vi "_Counter-Decrement.vi"(6 "LIBNAME":string, 7 "VI Refnum":refnum<vi>, 8 "error in (no error)":errorcluster, 9 "force destroy?(F)":bool, 11 "StopSignal":T2) -> (0 "error out":errorcluster, 1 "cache":T1)   [LabVIEW 2017, in "StopSignal.lvlib"]
uses:
  StopSignal.lvlib
  Typedef/StopSignal.ctl
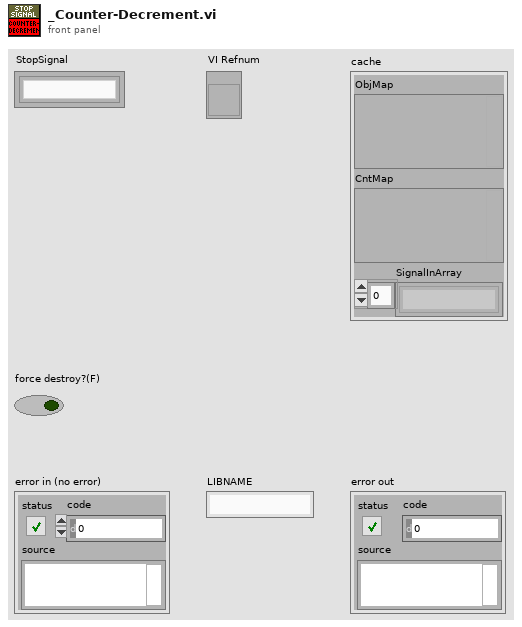
[diagram p1: front panel]
types:
  T1 = cluster{"ObjMap":variant, "CntMap":variant, "SignalInArray":string[]}
  T2 = typedef "StopSignal.lvlib/StopSignal.ctl" = refnum<k1>
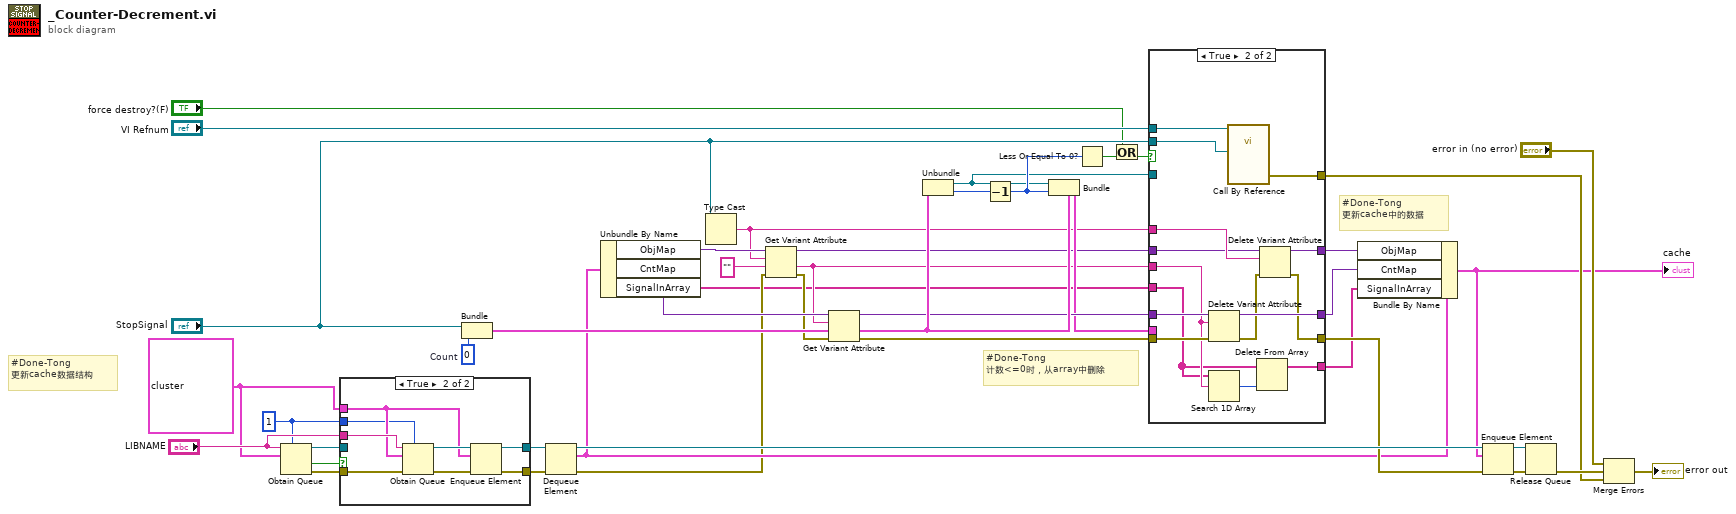
[diagram p0: block diagram]
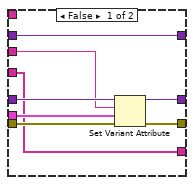
[diagram p2: hidden frame]
diagram:
  w4 = T1 {"ObjMap"=variant, "CntMap"=variant, "SignalInArray"=[]}
  w20 = 1 ("max queue size (-1, unlimited)")
  w30 = 0  # Count
  # "#Done-Tong\n更新cache中的数据"
  # "#Done-Tong\n计数<=0时，从array中删除"
  # "#Done-Tong\n更新cache数据结构"
  n1 = Obtain Queue(max queue size (-1, unlimited)=w20, name (unnamed)="LIBNAME", element data type=w4) -> (queue out=w41:refnum<queue>, created new?=w43:bool, error out=w42:errorcluster)  [unwired: 2 in]
  n2 = case shown="True" w43 {
    tunnel: w42 -> [w45 w52]
    tunnel: w41 -> [w46 _]
    tunnel: w4 -> [_ w48]
    tunnel: [w45 w54] -> w40
    tunnel: [w46 w53] -> w39
    tunnel: "LIBNAME" -> [_ w49]
    tunnel: w20 -> [_ w47]
    frame False {
    }
    frame True {
      n3 = Obtain Queue(max queue size (-1, unlimited)=w47, name (unnamed)=w49, element data type=w48, error in (no error)=w52) -> (queue out=w50:refnum<queue>, error out=w51:errorcluster)  [unwired: 1 in, 1 out]
      n4 = Enqueue Element(queue=w50, element=w48, error in (no error)=w51) -> (queue out=w53:refnum<queue>, error out=w54:errorcluster)  [unwired: 1 in, 1 out]
    }
  }
  n5 = Bundle("StopSignal"="StopSignal", "Count"=w30) -> (w29:cluster{"StopSignal":T2, "Count":i32})  [unwired: 1 in]
  n6 = Dequeue Element(queue=w39, error in (no error)=w40) -> (queue out=w35:refnum<queue>, element=w18:T1, error out=w9:errorcluster)  [unwired: 1 in, 1 out]
  n7 = Unbundle By Name(w18) -> ("ObjMap"=w15:variant, "CntMap"=w19:variant, "SignalInArray"=w3:string[])
  n8 = Type Cast(x="StopSignal") -> (*(type *) &x=w10:string)  [unwired: 1 in]
  n9 = Get Variant Attribute(Variant=w15, name=w10, default value (empty Variant)="" ("type"), error in=w9) -> (duplicate Variant=w12:variant, value=w11:string, error out=w8:errorcluster)  [unwired: 1 out]
  n10 = Get Variant Attribute(Variant=w19, name=w11, default value (empty Variant)=w29, error in=w8) -> (duplicate Variant=w37:variant, value=w38:cluster{"StopSignal":T2, "Count":i32}, error out=w32:errorcluster)  [unwired: 1 out]
  n11 = Unbundle(w38) -> ("StopSignal"=w22:T2, "Count"=w25:i32)
  n12 = Decrement(x=w25) -> (x-1=w24:i32)
  n13 = Bundle(cluster=w38, "StopSignal"=w22, "Count"=w24) -> (w36:cluster{"StopSignal":T2, "Count":i32})
  n14 = Less Or Equal To 0?(x=w24) -> (x <= 0?=w6:bool)
  n15 = Or(x="force destroy?(F)", y=w6) -> (x .or. y?=w5:bool)
  n16 = case shown="True" w5 {
    tunnel: [w62 w76] -> w17
    tunnel: w37 -> [w61 w77]
    tunnel: w36 -> [w60 _]
    tunnel: w32 -> [w59 w75]
    tunnel: [w58 w67] -> w31
    tunnel: w11 -> [w57 w66]
    tunnel: "VI Refnum" -> [_ w74]
    tunnel: w22 -> [_ _]
    tunnel: [_ w73] -> w21
    tunnel: "StopSignal" -> [_ w72]
    tunnel: [w56 w69] -> w13
    tunnel: w12 -> [w56 w70]
    tunnel: w10 -> [_ w71]
    tunnel: w3 -> [w55 w64]
    tunnel: [w55 w63] -> w2
    frame False {
      n17 = Set Variant Attribute(Variant=w61, name=w57, value=w60, error in=w59) -> (Variant out=w62:variant, error out=w58:errorcluster)  [unwired: 1 out]
    }
    frame True {
      n18 = Delete Variant Attribute(4:w75, 6:w66, 7:w77) -> (0:w68:errorcluster, 3:w76:variant)  [unwired: 1 out]
      n19 = Search 1D Array(1D array=w64, element=w66) -> (index of element=w65:i32)  [unwired: 1 in]
      n20 = call-by-ref "?"(reference=w74, "StopSignal"=w72) -> ("error out"=w73:errorcluster)  [unwired: 11 in, 2 out]
      n21 = Delete From Array(array=w64, index=w65) -> (array with subset deleted=w63:string[])  [unwired: 1 in, 1 out]
      n22 = Delete Variant Attribute(4:w68, 6:w71, 7:w70) -> (0:w67:errorcluster, 3:w69:variant)  [unwired: 1 out]
    }
  }
  n23 = Bundle By Name(cluster=w18, "ObjMap"=w13, "CntMap"=w17, "SignalInArray"=w2) -> (w1:T1)
  "cache" <- w1
  n24 = Enqueue Element(queue=w35, element=w1, error in (no error)=w31) -> (queue out=w34:refnum<queue>, error out=w33:errorcluster)  [unwired: 1 in, 1 out]
  n25 = Release Queue(queue=w34, error in (no error)=w33) -> (error out=w44:errorcluster)  [unwired: 1 in, 2 out]
  n26 = Merge Errors("error in (no error)", w44, w21) -> (→"error out":errorcluster)
